vi "synth_channel.vi"(8 "error in (no error)":errorcluster, 11 "Program Data":T1={"task ID"=0, "Data"=[], "Frequecies"=[], "Audio Settings"={"device ID"=0, "Buffer Size"=64.0, "sound format"={"sample rate (S/s)"=22050.0, "number of channels"=2, "bits per sample"=16}, "Number of samples"=0}, "Monitoring"={"Pressed Key Nr"=0, "Played Freqency"=0.0, "Max Amplitude"=0.0, "Current Amplitude"=0.0, "Played Freqency 2"=0.0, "Played Freqency drone"=0.0}, "Wave settings"={"HI freq"=0.0, "LOW freq"=0.0, "wave type"=enum."Sine", "Distortion level"=0.0, "MIX volume"=0.0, "wave type 2"=enum."Sine", "wave type drone"=enum."Sine", "DRONE volume 2"=0.0}} {"task ID" format="%.0x"}) -> (0 "error out":errorcluster, 2 "output wave 2":dbl[](array[numeric]), 3 "output wave":dbl[](array[numeric]))   [LabVIEW 2024]
uses:
  controls/#typedef_program_data.ctl
  <vilib>/sound2/lvsound2.llb/Sound Output Task ID.ctl
  controls/#typedef_audio_settings.ctl
  <vilib>/sound2/lvsound2.llb/Sound Data Format.ctl
  controls/#typedef_monitoring.ctl
  controls/#typedef_wave_settings.ctl
  controls/#typedef_wave_types.ctl
  <vilib>/Analysis/NI_AALBase.lvlib
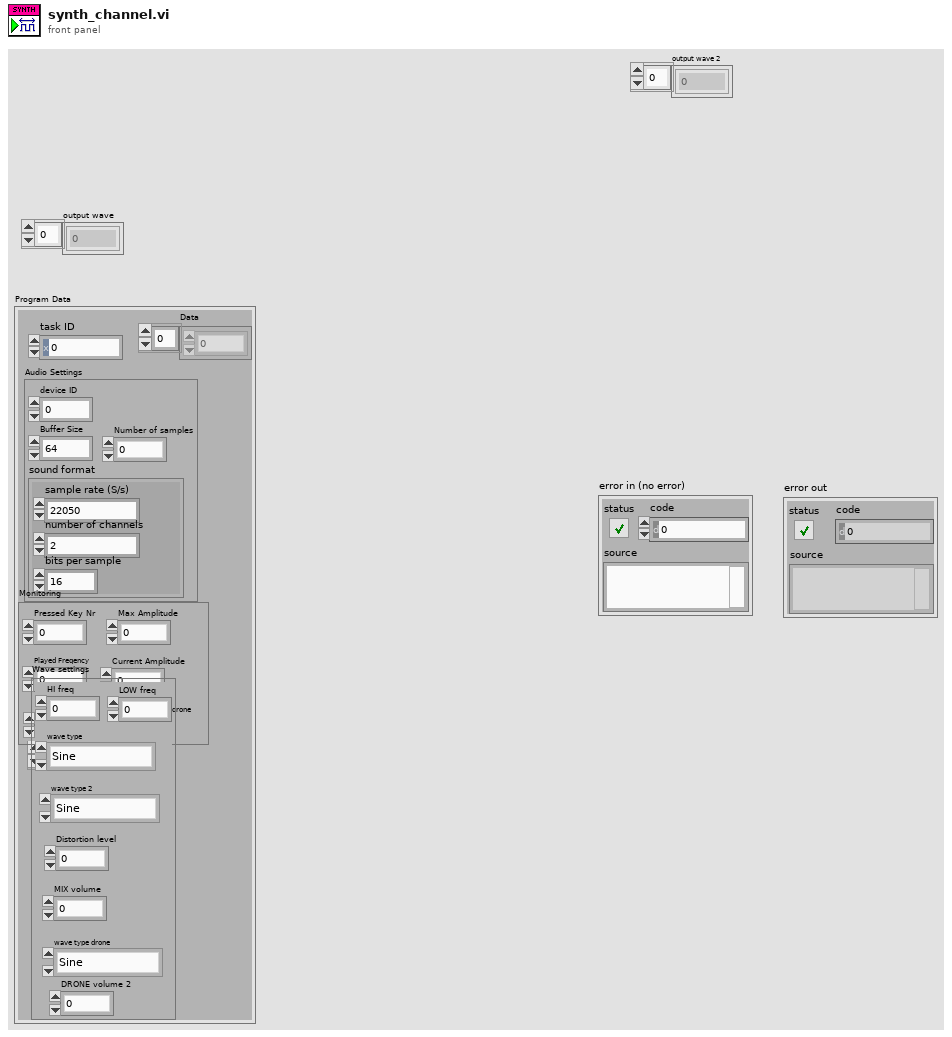
[diagram p1: front panel]
types:
  T1 = typedef "#typedef_program_data.ctl" = cluster{"task ID":T2, "Data":dbl[], "Frequecies":dbl[], "Audio Settings":T3, "Monitoring":T5, "Wave settings":T6}
  T2 = typedef "Sound Output Task ID.ctl" = u32
  T3 = typedef "#typedef_audio_settings.ctl" = cluster{"device ID":u32, "Buffer Size":dbl, "sound format":T4, "Number of samples":i32}
  T4 = typedef "Sound Data Format.ctl" = cluster{"sample rate (S/s)":dbl, "number of channels":i32, "bits per sample":i32}
  T5 = typedef "#typedef_monitoring.ctl" = cluster{"Pressed Key Nr":i32, "Played Freqency":dbl, "Max Amplitude":dbl, "Current Amplitude":dbl, "Played Freqency 2":dbl, "Played Freqency drone":dbl}
  T6 = typedef "#typedef_wave_settings.ctl" = cluster{"HI freq":dbl, "LOW freq":dbl, "wave type":T7, "Distortion level":dbl, "MIX volume":dbl, "wave type 2":T7, "wave type drone":T7, "DRONE volume 2":dbl}
  T7 = typedef "#typedef_wave_types.ctl" = enum16{"Sine", "Square", "Sawtooth", "Triangle"}
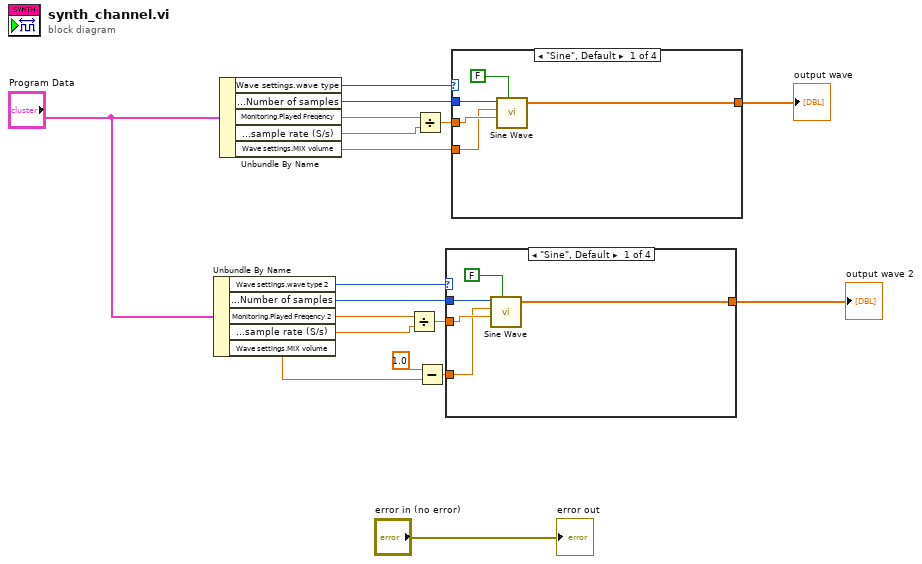
[diagram p0: block diagram]
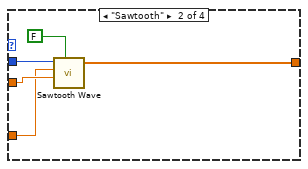
[diagram p2: hidden frame]
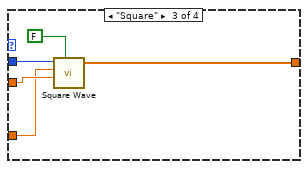
[diagram p3: hidden frame]
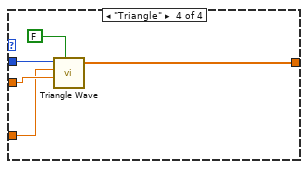
[diagram p4: hidden frame]
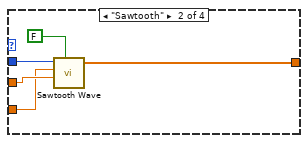
[diagram p5: hidden frame]
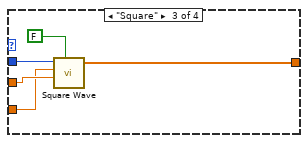
[diagram p6: hidden frame]
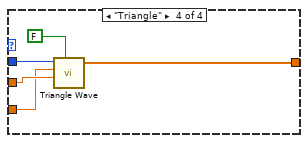
[diagram p7: hidden frame]
diagram:
  n1 = Unbundle By Name("Program Data") -> ("Wave settings.wave type 2"=w10:T7, "Audio Settings.Number of samples"=w9:i32, "Monitoring.Played Freqency 2"=w11:dbl, "Audio Settings.sound format.sample rate (S/s)"=w12:dbl, "Wave settings.MIX volume"=w4:dbl)
  n2 = Unbundle By Name("Program Data") -> ("Wave settings.wave type"=w15:T7, "Audio Settings.Number of samples"=w16:i32, "Monitoring.Played Freqency"=w14:dbl, "Audio Settings.sound format.sample rate (S/s)"=w13:dbl, "Wave settings.MIX volume"=w6:dbl)
  n3 = Divide(x=w11, y=w12) -> (x/y=w8:dbl)
  n4 = Divide(x=w14, y=w13) -> (x/y=w17:dbl)
  n5 = Subtract(x=1.0, y=w4) -> (x-y=w3:dbl)
  n6 = case shown="\"Sine\", Default" w10 {
    tunnel: w9 -> [w22 w27 w33 w38]
    tunnel: w8 -> [w21 w28 w31 w36]
    tunnel: [w20 w26 w30 w37] -> w7
    tunnel: w3 -> [w19 w24 w29 w34]
    frame "Sine", Default {
      n7 = call <vilib>:"Sine Wave.vi"("samples"=w22, "amplitude"=w19, "frequency"=w21, "reset phase"=FALSE) -> ("sine wave"=w20:dbl[])  [unwired: 1 in, 2 out]
    }
    frame "Sawtooth" {
      n8 = call <vilib>:"Sawtooth Wave.vi"("samples"=w27, "amplitude"=w24, "frequency"=w28, "reset phase"=FALSE) -> ("sawtooth wave"=w26:dbl[])  [unwired: 1 in, 2 out]
    }
    frame "Square" {
      n9 = call <vilib>:"Square Wave.vi"("samples"=w33, "reset phase"=FALSE, "amplitude"=w29, "frequency"=w31) -> ("square wave"=w30:dbl[])  [unwired: 2 in, 2 out]
    }
    frame "Triangle" {
      n10 = call <vilib>:"Triangle Wave.vi"("samples"=w38, "amplitude"=w34, "frequency"=w36, "reset phase"=FALSE) -> ("triangle wave"=w37:dbl[])  [unwired: 1 in, 2 out]
    }
  }
  "output wave 2" <- w7
  n11 = case shown="\"Sine\", Default" w15 {
    tunnel: w16 -> [w42 w47 w53 w58]
    tunnel: w17 -> [w41 w48 w51 w56]
    tunnel: [w40 w46 w50 w57] -> w18
    tunnel: w6 -> [w39 w44 w49 w54]
    frame "Sine", Default {
      n12 = call <vilib>:"Sine Wave.vi"("samples"=w42, "amplitude"=w39, "frequency"=w41, "reset phase"=FALSE) -> ("sine wave"=w40:dbl[])  [unwired: 1 in, 2 out]
    }
    frame "Sawtooth" {
      n13 = call <vilib>:"Sawtooth Wave.vi"("samples"=w47, "amplitude"=w44, "frequency"=w48, "reset phase"=FALSE) -> ("sawtooth wave"=w46:dbl[])  [unwired: 1 in, 2 out]
    }
    frame "Square" {
      n14 = call <vilib>:"Square Wave.vi"("samples"=w53, "reset phase"=FALSE, "amplitude"=w49, "frequency"=w51) -> ("square wave"=w50:dbl[])  [unwired: 2 in, 2 out]
    }
    frame "Triangle" {
      n15 = call <vilib>:"Triangle Wave.vi"("samples"=w58, "amplitude"=w54, "frequency"=w56, "reset phase"=FALSE) -> ("triangle wave"=w57:dbl[])  [unwired: 1 in, 2 out]
    }
  }
  "output wave" <- w18
  "error out" <- "error in (no error)"
